vi "Test Insertion Palette Drag Drop.vi"   [LabVIEW 2020]
uses:
  TSnax UI/Basic UI State.ctl
  TSnax/Engine/TS License Type.ctl
  TSnax UI/SequenceViewPanel/SequenceViewPanel.lvclass
  TSnax UI/InsertionPalettePanel/InsertionPalettePanel.lvclass
  TSnax UI/TSnax UI Manager/TSnax UI Manager.lvclass
  TSnax/SequenceFile/SequenceFile.lvclass
  TSnax UI/TSnax UI.lvlib
  TSnax/Engine/Engine.lvclass
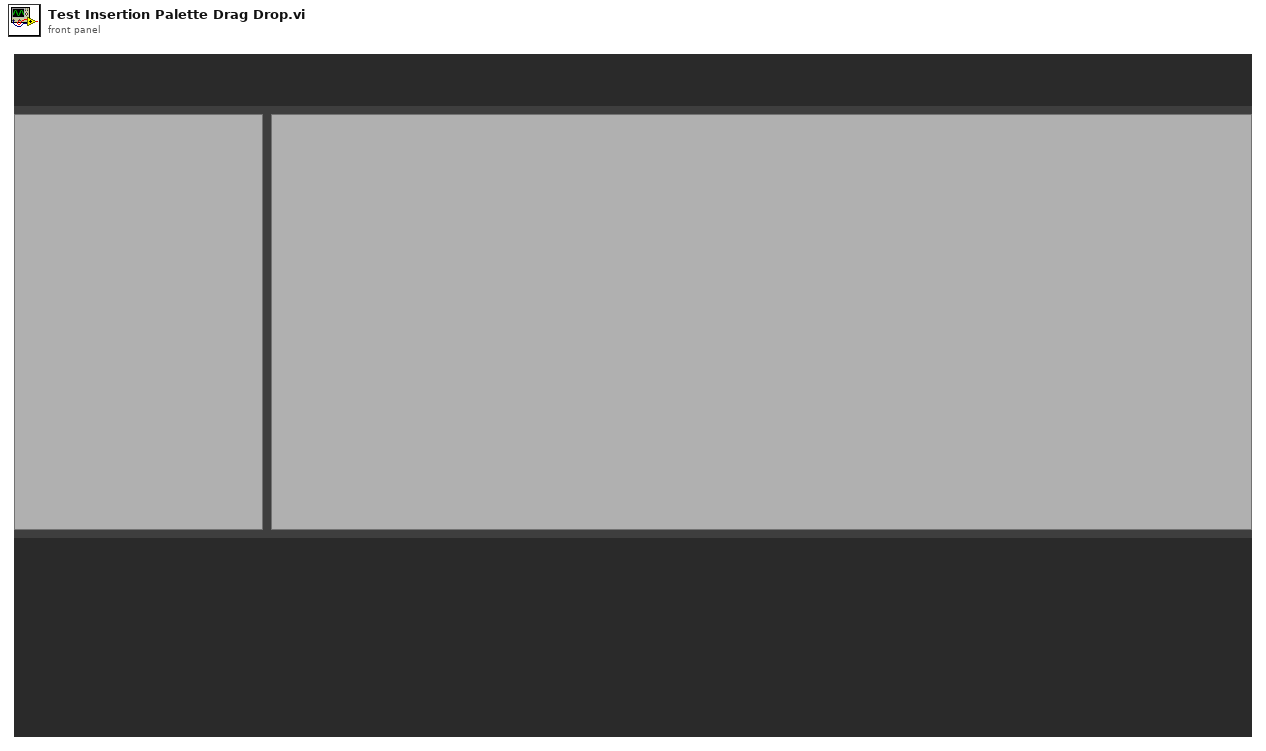
[diagram p1: front panel]
types:
  T1 = typedef "TSnax UI.lvlib/Basic UI State.ctl" = enum16{"Init", "Run", "Close"}
  T2 = typedef "TSnax.lvlib/Engine.lvclass/TS License Type.ctl" = enum16{"Operator", "CustomEditor", "SequenceEditor"}
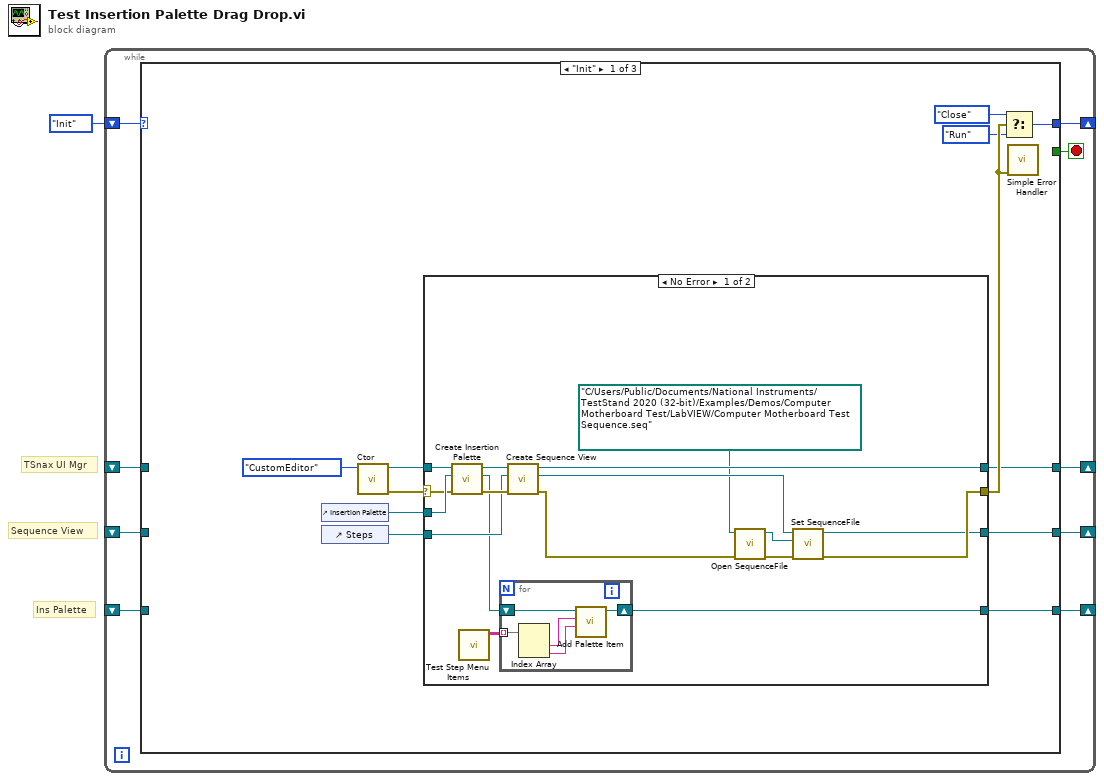
[diagram p0: block diagram]
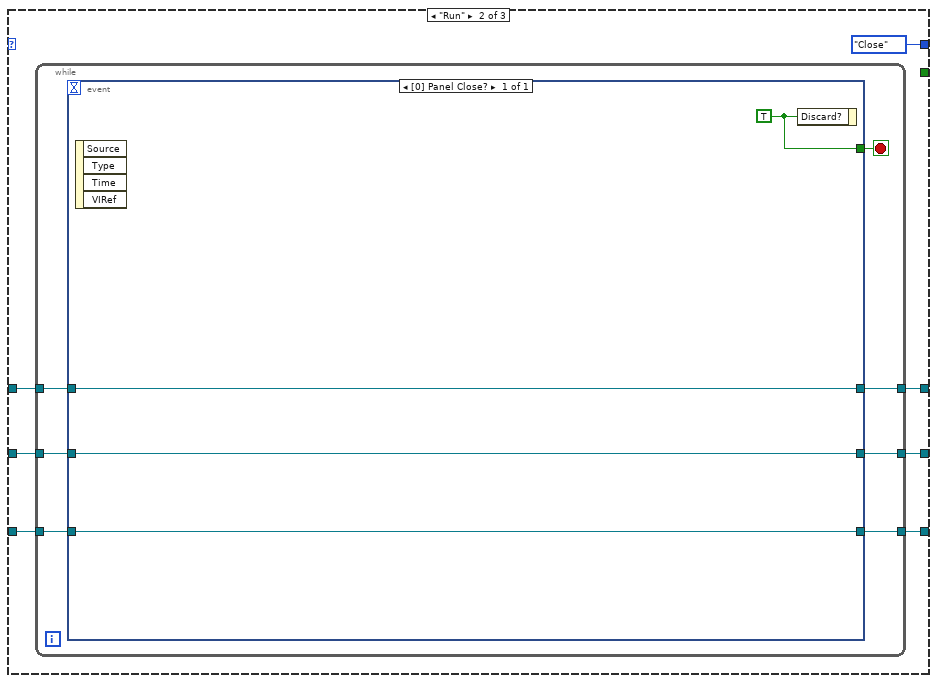
[diagram p3: hidden frame]
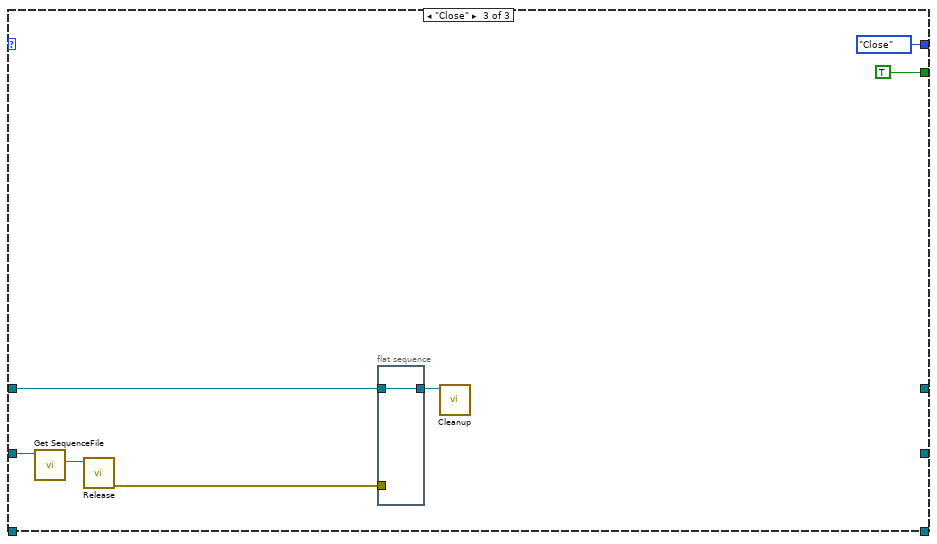
[diagram p4: hidden frame]
diagram:
  # "Ins Palette"
  # "Sequence View"
  # "TSnax UI Mgr"
  n1 = while {
    shift-right: [w9] -> _
    shift-left: Basic_UI_State."Init" ("Basic UI State") -> [w10]
    shift-right: [w7] -> _
    shift-left: _ -> [w6]
    shift-right: [w5] -> _
    shift-left: _ -> [w4]
    shift-right: [w3] -> _
    shift-left: _ -> [w2]
    stop <- w8 stop-if-true
    n2 = case shown="\"Init\"" w10 {
      tunnel: [w17 Basic_UI_State."Close" ("Basic UI State") Basic_UI_State."Close" ("Basic UI State")] -> w9
      tunnel: [_ _ TRUE] -> w8
      tunnel: [w15 w49 _] -> w7
      tunnel: w6 -> [_ w52 w66]
      tunnel: [w16 w48 _] -> w5
      tunnel: w4 -> [_ w51 w69]
      tunnel: [w21 w47 _] -> w3
      tunnel: w2 -> [_ w50 _]
      frame "Init" {
        n3 = control-ref of="Insertion Palette"() -> (w13:refnum<vi>)
        n4 = control-ref of="Steps"() -> (w14:refnum<vi>)
        n5 = call "Ctor.vi"("TS License Type (Operator)"=TS_License_Type."CustomEditor") -> ("error out"=w11:errorcluster, "TSnax UI Manager out"=w12:refnum<class "TSnax UI Manager.lvclass">)  [unwired: 8 in, 1 out]
        n6 = case shown="No Error" w11 {
          selector: w11 -> [w32 w45]
          tunnel: [w39 _] -> w21
          tunnel: w12 -> [w33 w46]
          tunnel: [w27 _] -> w16
          tunnel: [w30 w46] -> w15
          tunnel: w14 -> [w35 _]
          tunnel: w13 -> [w34 _]
          tunnel: [w28 w45] -> w22
          frame No Error {
            n7 = call "Create Insertion Palette.vi"("error in (no error)"=w32, "Subpanel"=w34, "TSnax UI Manager in"=w33) -> ("error out"=w36:errorcluster, "Insertion Palette"=w31:refnum<class "InsertionPalettePanel.lvclass">, "TSnax UI Manager out"=w37:refnum<class "TSnax UI Manager.lvclass">)  [unwired: 6 in]
            n8 = call "Test Step Menu Items.vi"() -> ("Array"=w38:string[][])  [unwired: 11 in]
            n9 = for {
              shift-right: [w43] -> w39
              shift-left: w31 -> [w44]
              tunnel: w38 -> [w42] mode=indexing
              n10 = Index Array(array=w42) -> (element #1=w41:string, element #2=w40:string)  [unwired: 2 in]
              n11 = call "Add Palette Item.vi"("Group (From Step Type)"=w40, "Step Type Name"=w41, "InsertionPalettePanel in"=w44) -> ("InsertionPalettePanel out"=w43:refnum<class "InsertionPalettePanel.lvclass">)  [unwired: 7 in, 1 out]
            }
            n12 = call "Create Sequence View.vi"("error in (no error)"=w36, "Subpanel"=w35, "TSnax UI Manager in"=w37) -> ("error out"=w25:errorcluster, "Sequence View"=w29:refnum<class "SequenceViewPanel.lvclass">, "TSnax UI Manager out"=w30:refnum<class "TSnax UI Manager.lvclass">)  [unwired: 6 in]
            n13 = call "Open SequenceFile.vi"("error in (no error)"=w25, "Path"=path "C:/Users/Public/Documents/National Instruments/TestStand 2020 (32-bit)/Examples/Demos/Computer Motherboard Test/LabVIEW/Computer Motherboard Test Sequence.seq") -> ("error out"=w24:errorcluster, "SequenceFile out"=w23:refnum<class "SequenceFile.lvclass">)  [unwired: 8 in]
            n14 = call "Set SequenceFile.vi"("error in (no error)"=w24, "SequenceFile"=w23, "SequenceViewPanel in"=w29) -> ("error out"=w28:errorcluster, "SequenceViewPanel out"=w27:refnum<class "SequenceViewPanel.lvclass">)  [unwired: 7 in]
          }
          frame Error {
          }
        }
        n15 = Select(t=Basic_UI_State."Close" ("Basic UI State"), s=w22, f=Basic_UI_State."Run") -> (s? t:f=w17:T1)
        n16 = call <vilib>:"Simple Error Handler.vi"("error in (no error)"=w22) -> ()  [unwired: 4 in, 5 out]
      }
      frame "Run" {
        n17 = while {
          tunnel: w52 -> [w60]
          tunnel: w51 -> [w59]
          tunnel: w50 -> [w58]
          tunnel: [w56] -> w49
          tunnel: [w55] -> w48
          tunnel: [w54] -> w47
          stop <- w57 stop-if-true
          n18 = event shown="[0] Panel Close?" {
            selector: _ -> [_]
            dyn-events: _ -> [_]
            timeout: _ -> [_]
            tunnel: w60 -> [w63]
            tunnel: w59 -> [w62]
            tunnel: w58 -> [w61]
            tunnel: [w64] -> w57
            tunnel: [w63] -> w56
            tunnel: [w62] -> w55
            tunnel: [w61] -> w54
            event Panel Close? {
              w64 = TRUE ("Discard?")
              n19 = event-data() -> ()  [unwired: 1 in, 4 out]
              n20 = event-data("Discard?"=w64) -> ()  [unwired: 1 in, 1 out]
            }
          }
        }
      }
      frame "Close" {
        n21 = call "Get SequenceFile.vi"("SequenceViewPanel in"=w69) -> ("SequenceFile"=w68:refnum<class "SequenceFile.lvclass">)  [unwired: 8 in, 2 out]
        n22 = call-dynamic "Release.vi"("SequenceFile in"=w68) -> ("error out"=w67:errorcluster)  [unwired: 10 in]
        n23 = flat-sequence {
          tunnel: w67 -> [_]
          tunnel: w66 -> [w72]
          tunnel: [w72] -> w65
          frame #0 {
          }
        }
        n24 = call "Cleanup.vi"("TSnax UI Manager in"=w65) -> ()  [unwired: 10 in, 1 out]
      }
    }
  }
